vi "CalculateLowUpdateDeviceFeatures.vi"(8 "error in (no error)":errorcluster, 9 "data flow map in":T11, 10 "Waveforms":waveform(sgl)[](array[waveform]), 11 "Group in":T1={"Name"="", "Channels"=[], "Motor Information"={"Model"="", "Manufacturer"="", "Serial Number"="", "Horsepower"=0.0, "Horsepower Unit"="", "Full Load Speed"=0.0, "Synchronous Speed"=0.0, "Rated Volts"=0.0, "Full Load Amps"=0.0, "Frequency"=0.0, "Service Factor"=0.0, "Efficiency"=0.0, "Efficiency @ 75% Load"=0.0, "Efficiency @ 50% Load"=0.0, "Efficiency @ 25% Load"=0.0, "Power Factor"=0.0, "VoltageBus"="", "VoltageBus ID"="", "Stator Resistance"=0.0, "Estimate Stator Resistance"=FALSE}, "Calculation Cache"={"Spectrum Reset"=FALSE, "Spectrum"={"f0"=0.0, "df"=0.0, "magnitude [dB]"=[]}, "max sideband magnitude [dB]"=-100.0, "rotor sideband step [Hz]"=0.0, "spectrum initial conditions"={"hilbert state"={"delay conditions"=[], "filter conditions"=[]}, "zoom FFT state"={"phase state"=0.0, "zoom FFT state"={"zoom settings state"={"zoom"=0, "stop band attenuation"=enum."84 dB", "alias protect in final transition"=FALSE, "oversampling ratio"=0.0}, "SML Decimation Filter (complex input) state"={"decimation settings state"={"M"=0, "stop band attenuation"=enum."84 dB", "alias protect in transition band"=FALSE, "oversampling ratio"=0.0}, "counter for garbage samples state"=0, "sml_Parameter Setting for Zoom Factor state"={"filter length * interpolation state"=0, "interpolation state"=0, "comb filter order state"=0, "CFIR par state"={"h"=[], "M"=0, "N"=0}, "LFIR par state"={"h"=[], "M"=0, "N"=0}, "CIC Stages state"=0}, "aal_CIC (complex input) state"={"aal_cascaded moving average (complex input) state"={"states"=[], "circular buffers state"=[], "circular buffer counter state"=0}, "aal_moving average with decimation by order (complex input) state"={"residue result state"=0.0+0.0i, "processed data counter state"=0}}, "sml_Cascaded Decimation Filter (complex input) CFIR state"={"unprocessed data state"=[], "final conditions state"=[], "sml_M-1 Decimator with IC (complex input) state"={"coefficients in reverse order state"=[], "max index for coefficients state"=0}}, "sml_Cascaded Decimation Filter (complex input) LFIR state"={"unprocessed data state"=[], "final conditions state"=[], "sml_M-1 Decimator with IC (complex input) state"={"coefficients in reverse order state"=[], "max index for coefficients state"=0}}}, "ma_SML Data Packing (complex input) state"={"array getting packed state"=[], "last array processed state"=[], "index state"=0, "packing parameters state"={0, "size"=0}}}, "FFT{X} [Vrms]"=[]}, "IIR filter state"={"filter state"=[]}, "demodulation settings"={"enable? (F)"=FALSE, "algorithm"=enum."1-phase signal"}, "highpass IIR Filter"={"filter structure"=enum."IIR 2nd Order", "Reverse Coefficients"=[], "Forward Coefficients"=[]}, "Hilbert FIR filter"={"coefficients"=[], "delay"=0}, "zoom FFT settings"={"FFT settings"={"window"=0, "Window Size"=0, "FFT Size"=0, "%overlap"=0.0}, "zoom settings"={"zoom"=0, "stop band attenuation"=enum."84 dB", "alias protect in final transition"=FALSE, "oversampling ratio"=0.0}, "other settings"={"fmod"=0.0, "f0"=0.0, "df"=0.0, "oidx"=0, "olen"=0}, "iterations"=0, "max block size"=0, "fs"=0.0}}, "Speed Reset"=FALSE, "speed [RPM]"=0.0, "slip"=0.0, "speed initial conditions"={"SVAF state"={"space vector amplitude"=0.0, "hilbert state"={"delay conditions"=[], "filter conditions"=[]}}, "zoom FFT state"={"phase state"=0.0, "zoom FFT state"={"zoom settings state"={"zoom"=0, "stop band attenuation"=enum."84 dB", "alias protect in final transition"=FALSE, "oversampling ratio"=0.0}, "SML Decimation Filter (complex input) state"={"decimation settings state"={"M"=0, "stop band attenuation"=enum."84 dB", "alias protect in transition band"=FALSE, "oversampling ratio"=0.0}, "counter for garbage samples state"=0, "sml_Parameter Setting for Zoom Factor state"={"filter length * interpolation state"=0, "interpolation state"=0, "comb filter order state"=0, "CFIR par state"={"h"=[], "M"=0, "N"=0}, "LFIR par state"={"h"=[], "M"=0, "N"=0}, "CIC Stages state"=0}, "aal_CIC (complex input) state"={"aal_cascaded moving average (complex input) state"={"states"=[], "circular buffers state"=[], "circular buffer counter state"=0}, "aal_moving average with decimation by order (complex input) state"={"residue result state"=0.0+0.0i, "processed data counter state"=0}}, "sml_Cascaded Decimation Filter (complex input) CFIR state"={"unprocessed data state"=[], "final conditions state"=[], "sml_M-1 Decimator with IC (complex input) state"={"coefficients in reverse order state"=[], "max index for coefficients state"=0}}, "sml_Cascaded Decimation Filter (complex input) LFIR state"={"unprocessed data state"=[], "final conditions state"=[], "sml_M-1 Decimator with IC (complex input) state"={"coefficients in reverse order state"=[], "max index for coefficients state"=0}}}, "ma_SML Data Packing (complex input) state"={"array getting packed state"=[], "last array processed state"=[], "index state"=0, "packing parameters state"={0, "size"=0}}}, "FFT{X} [Vrms]"=[]}, "speed state"={"speed [RPM]"=0.0, "slip"=0.0}, "speed estimation settings"={"% overlap"=0.0, "algorithm"=enum."1-phase signal"}, "filter information"={"coefficients"=[], "order"=0}, "zoom FFT settings"={"FFT settings"={"window"=0, "Window Size"=0, "FFT Size"=0, "%overlap"=0.0}, "zoom settings"={"zoom"=0, "stop band attenuation"=enum."84 dB", "alias protect in final transition"=FALSE, "oversampling ratio"=0.0}, "other settings"={"fmod"=0.0, "f0"=0.0, "df"=0.0, "oidx"=0, "olen"=0}, "iterations"=0, "max block size"=0, "fs"=0.0}, "last valid window"=0, "fund. frequency for averager"=[]}, "line frequency [Hz]"=0.0}} {"Calculation Cache"."speed initial conditions"."zoom FFT settings"."FFT settings"."window" items=["Rectangle"=0, "Hanning"=1, "Hamming"=2, "Blackman-Harris"=3, "Exact Blackman"=4, "Blackman"=5, "Flat Top"=6, "4 Term B-Harris "=7, "7 Term B-Harris"=8, "Low Sidelobe"=9, "Blackman Nuttall"=11, "Triangle"=30, "Bartlett-Hanning"=31, "Bohman"=32, "Parzen"=33, "Welch"=34, "Kaiser"=60, "Dolph-Chebyshev"=61, "Gaussian"=62]; "Calculation Cache"."spectrum initial conditions"."zoom FFT settings"."FFT settings"."window" items=["Rectangle"=0, "Hanning"=1, "Hamming"=2, "Blackman-Harris"=3, "Exact Blackman"=4, "Blackman"=5, "Flat Top"=6, "4 Term B-Harris "=7, "7 Term B-Harris"=8, "Low Sidelobe"=9, "Blackman Nuttall"=11, "Triangle"=30, "Bartlett-Hanning"=31, "Bohman"=32, "Parzen"=33, "Welch"=34, "Kaiser"=60, "Dolph-Chebyshev"=61, "Gaussian"=62]}) -> (0 "error out":errorcluster, 3 "Group out":T1={"Name"="", "Channels"=[], "Motor Information"={"Model"="", "Manufacturer"="", "Serial Number"="", "Horsepower"=0.0, "Horsepower Unit"="", "Full Load Speed"=0.0, "Synchronous Speed"=0.0, "Rated Volts"=0.0, "Full Load Amps"=0.0, "Frequency"=0.0, "Service Factor"=0.0, "Efficiency"=0.0, "Efficiency @ 75% Load"=0.0, "Efficiency @ 50% Load"=0.0, "Efficiency @ 25% Load"=0.0, "Power Factor"=0.0, "VoltageBus"="", "VoltageBus ID"="", "Stator Resistance"=0.0, "Estimate Stator Resistance"=FALSE}, "Calculation Cache"={"Spectrum Reset"=FALSE, "Spectrum"={"f0"=0.0, "df"=0.0, "magnitude [dB]"=[]}, "max sideband magnitude [dB]"=-100.0, "rotor sideband step [Hz]"=0.0, "spectrum initial conditions"={"hilbert state"={"delay conditions"=[], "filter conditions"=[]}, "zoom FFT state"={"phase state"=0.0, "zoom FFT state"={"zoom settings state"={"zoom"=0, "stop band attenuation"=enum."84 dB", "alias protect in final transition"=FALSE, "oversampling ratio"=0.0}, "SML Decimation Filter (complex input) state"={"decimation settings state"={"M"=0, "stop band attenuation"=enum."84 dB", "alias protect in transition band"=FALSE, "oversampling ratio"=0.0}, "counter for garbage samples state"=0, "sml_Parameter Setting for Zoom Factor state"={"filter length * interpolation state"=0, "interpolation state"=0, "comb filter order state"=0, "CFIR par state"={"h"=[], "M"=0, "N"=0}, "LFIR par state"={"h"=[], "M"=0, "N"=0}, "CIC Stages state"=0}, "aal_CIC (complex input) state"={"aal_cascaded moving average (complex input) state"={"states"=[], "circular buffers state"=[], "circular buffer counter state"=0}, "aal_moving average with decimation by order (complex input) state"={"residue result state"=0.0+0.0i, "processed data counter state"=0}}, "sml_Cascaded Decimation Filter (complex input) CFIR state"={"unprocessed data state"=[], "final conditions state"=[], "sml_M-1 Decimator with IC (complex input) state"={"coefficients in reverse order state"=[], "max index for coefficients state"=0}}, "sml_Cascaded Decimation Filter (complex input) LFIR state"={"unprocessed data state"=[], "final conditions state"=[], "sml_M-1 Decimator with IC (complex input) state"={"coefficients in reverse order state"=[], "max index for coefficients state"=0}}}, "ma_SML Data Packing (complex input) state"={"array getting packed state"=[], "last array processed state"=[], "index state"=0, "packing parameters state"={0, "size"=0}}}, "FFT{X} [Vrms]"=[]}, "IIR filter state"={"filter state"=[]}, "demodulation settings"={"enable? (F)"=FALSE, "algorithm"=enum."1-phase signal"}, "highpass IIR Filter"={"filter structure"=enum."IIR 2nd Order", "Reverse Coefficients"=[], "Forward Coefficients"=[]}, "Hilbert FIR filter"={"coefficients"=[], "delay"=0}, "zoom FFT settings"={"FFT settings"={"window"=0, "Window Size"=0, "FFT Size"=0, "%overlap"=0.0}, "zoom settings"={"zoom"=0, "stop band attenuation"=enum."84 dB", "alias protect in final transition"=FALSE, "oversampling ratio"=0.0}, "other settings"={"fmod"=0.0, "f0"=0.0, "df"=0.0, "oidx"=0, "olen"=0}, "iterations"=0, "max block size"=0, "fs"=0.0}}, "Speed Reset"=FALSE, "speed [RPM]"=0.0, "slip"=0.0, "speed initial conditions"={"SVAF state"={"space vector amplitude"=0.0, "hilbert state"={"delay conditions"=[], "filter conditions"=[]}}, "zoom FFT state"={"phase state"=0.0, "zoom FFT state"={"zoom settings state"={"zoom"=0, "stop band attenuation"=enum."84 dB", "alias protect in final transition"=FALSE, "oversampling ratio"=0.0}, "SML Decimation Filter (complex input) state"={"decimation settings state"={"M"=0, "stop band attenuation"=enum."84 dB", "alias protect in transition band"=FALSE, "oversampling ratio"=0.0}, "counter for garbage samples state"=0, "sml_Parameter Setting for Zoom Factor state"={"filter length * interpolation state"=0, "interpolation state"=0, "comb filter order state"=0, "CFIR par state"={"h"=[], "M"=0, "N"=0}, "LFIR par state"={"h"=[], "M"=0, "N"=0}, "CIC Stages state"=0}, "aal_CIC (complex input) state"={"aal_cascaded moving average (complex input) state"={"states"=[], "circular buffers state"=[], "circular buffer counter state"=0}, "aal_moving average with decimation by order (complex input) state"={"residue result state"=0.0+0.0i, "processed data counter state"=0}}, "sml_Cascaded Decimation Filter (complex input) CFIR state"={"unprocessed data state"=[], "final conditions state"=[], "sml_M-1 Decimator with IC (complex input) state"={"coefficients in reverse order state"=[], "max index for coefficients state"=0}}, "sml_Cascaded Decimation Filter (complex input) LFIR state"={"unprocessed data state"=[], "final conditions state"=[], "sml_M-1 Decimator with IC (complex input) state"={"coefficients in reverse order state"=[], "max index for coefficients state"=0}}}, "ma_SML Data Packing (complex input) state"={"array getting packed state"=[], "last array processed state"=[], "index state"=0, "packing parameters state"={0, "size"=0}}}, "FFT{X} [Vrms]"=[]}, "speed state"={"speed [RPM]"=0.0, "slip"=0.0}, "speed estimation settings"={"% overlap"=0.0, "algorithm"=enum."1-phase signal"}, "filter information"={"coefficients"=[], "order"=0}, "zoom FFT settings"={"FFT settings"={"window"=0, "Window Size"=0, "FFT Size"=0, "%overlap"=0.0}, "zoom settings"={"zoom"=0, "stop band attenuation"=enum."84 dB", "alias protect in final transition"=FALSE, "oversampling ratio"=0.0}, "other settings"={"fmod"=0.0, "f0"=0.0, "df"=0.0, "oidx"=0, "olen"=0}, "iterations"=0, "max block size"=0, "fs"=0.0}, "last valid window"=0, "fund. frequency for averager"=[]}, "line frequency [Hz]"=0.0}} {"Calculation Cache"."speed initial conditions"."zoom FFT settings"."FFT settings"."window" items=["Rectangle"=0, "Hanning"=1, "Hamming"=2, "Blackman-Harris"=3, "Exact Blackman"=4, "Blackman"=5, "Flat Top"=6, "4 Term B-Harris "=7, "7 Term B-Harris"=8, "Low Sidelobe"=9, "Blackman Nuttall"=11, "Triangle"=30, "Bartlett-Hanning"=31, "Bohman"=32, "Parzen"=33, "Welch"=34, "Kaiser"=60, "Dolph-Chebyshev"=61, "Gaussian"=62]; "Calculation Cache"."spectrum initial conditions"."zoom FFT settings"."FFT settings"."window" items=["Rectangle"=0, "Hanning"=1, "Hamming"=2, "Blackman-Harris"=3, "Exact Blackman"=4, "Blackman"=5, "Flat Top"=6, "4 Term B-Harris "=7, "7 Term B-Harris"=8, "Low Sidelobe"=9, "Blackman Nuttall"=11, "Triangle"=30, "Bartlett-Hanning"=31, "Bohman"=32, "Parzen"=33, "Welch"=34, "Kaiser"=60, "Dolph-Chebyshev"=61, "Gaussian"=62]})   [LabVIEW 2017, in "McsaAnalysisLowUpdate.lvlib"]
uses:
  <vilib>/addons/InsightCM/Devices/Shared/Mcsa/McsaAnalysisLowUpdate/McsaAnalysisLowUpdate.lvlib
  <vilib>/addons/PointValueMap/controls/PointMap.ctl
  <vilib>/addons/InsightCM/Devices/Shared/Mcsa/McsaAnalysisLowUpdate/controls/Group.ctl
  <vilib>/addons/InsightCM/Utilities/Analysis/MCSA/controls/McsaLowUpdateChannel.ctl
  <vilib>/addons/InsightCM/Utilities/Analysis/Shared/controls/Feature.ctl
  <vilib>/addons/InsightCM/Utilities/Analysis/Shared/controls/AmplitudeScale.ctl
  <vilib>/addons/InsightCM/Utilities/Analysis/MCSA/controls/McsaMotor.ctl
  <vilib>/addons/InsightCM/Utilities/Analysis/MCSA/controls/McsaCalculationCache.ctl
  <vilib>/addons/Electrical Power/Motor Monitoring/subVIs/ep_Initial Conditions for MCSA Spectra.ctl
  <vilib>/addons/Electrical Power/Motor Monitoring/subVIs/ep_Demodulation Algorithm.ctl
  <vilib>/addons/Electrical Power/Motor Monitoring/subVIs/ep_Zoom FFT Settings.ctl
  <vilib>/addons/Electrical Power/Motor Monitoring/subVIs/ep_Initial Conditions for Speed Estimation.ctl
  <vilib>/addons/InsightCM/Utilities/Analysis/MCSA/McsaAnalysisFunctions.lvlib
  <vilib>/addons/PointValueMap/PointValueMap.lvlib
  <vilib>/addons/InsightCM/Utilities/Analysis/Shared/AnalysisHelper.lvlib
  <vilib>/addons/Electrical Power/Motor Monitoring/NI_EP_Motor Monitoring.lvlib
panel:
  out "data flow map out":T11
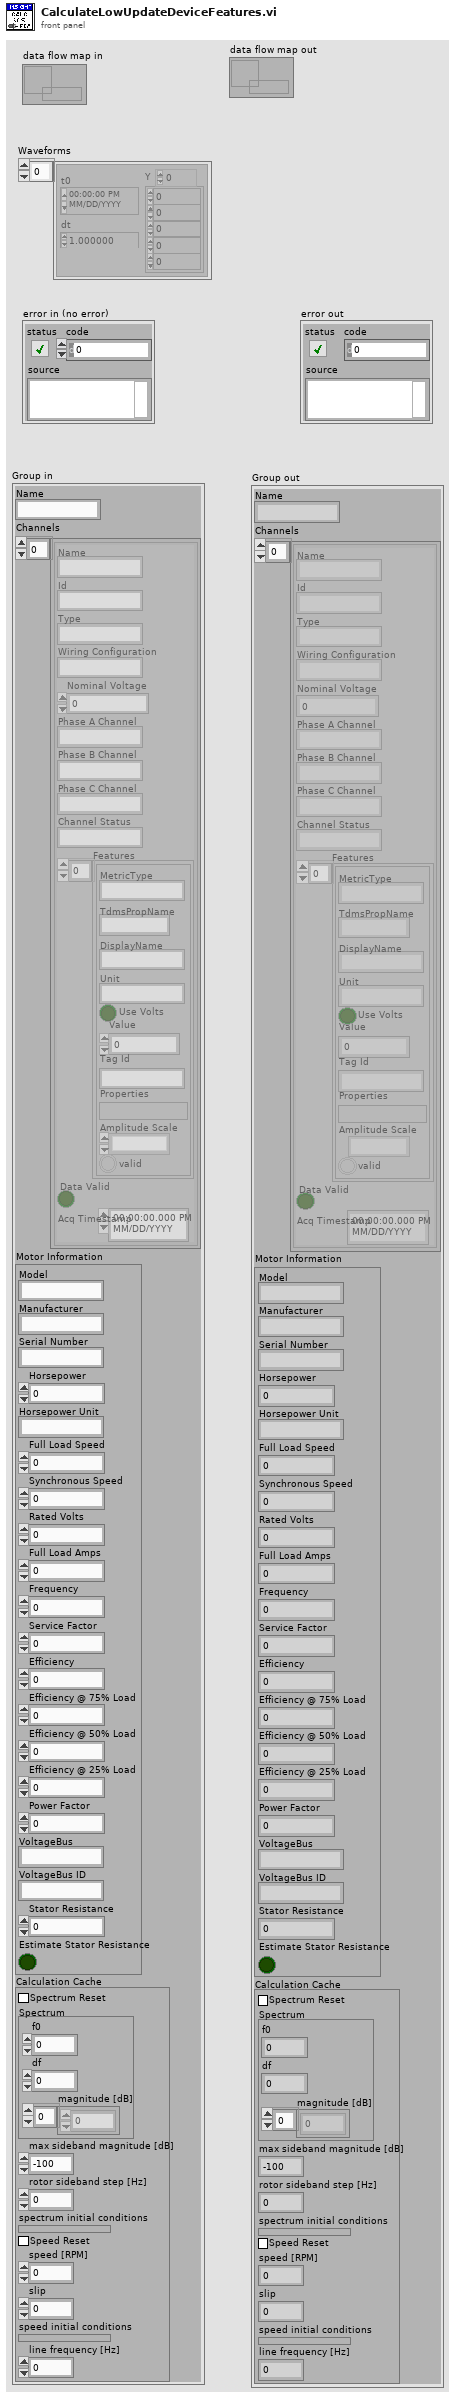
[diagram p1: front panel]
types:
  T1 = typedef "McsaAnalysisLowUpdate.lvlib/Group.ctl" = cluster{"Name":string, "Channels":T2[], "Motor Information":T5, "Calculation Cache":T6}
  T2 = typedef "McsaAnalysisFunctions.lvlib/McsaLowUpdateChannel.ctl" = cluster{"Name":string, "Id":string, "Type":string, "Wiring Configuration":string, "Nominal Voltage":dbl, "Phase A Channel":string, "Phase B Channel":string, "Phase C Channel":string, "Channel Status":string, "Features":T3[], "Data Valid":bool, "Acq Timestamp":timestamp}
  T3 = typedef "AnalysisHelper.lvlib/Feature.ctl" = cluster{"MetricType":string, "TdmsPropName":string, "DisplayName":string, "Unit":string, "Use Volts":bool, "Value":dbl, "Tag Id":string, "Properties":variant, "Amplitude Scale":T4, "valid":bool}
  T4 = typedef "AnalysisHelper.lvlib/AmplitudeScale.ctl" = enum16{"rms", "peak", "pk-pk"}
  T5 = typedef "McsaAnalysisFunctions.lvlib/McsaMotor.ctl" = cluster{"Model":string, "Manufacturer":string, "Serial Number":string, "Horsepower":dbl, "Horsepower Unit":string, "Full Load Speed":dbl, "Synchronous Speed":dbl, "Rated Volts":dbl, "Full Load Amps":dbl, "Frequency":dbl, "Service Factor":dbl, "Efficiency":dbl, "Efficiency @ 75% Load":dbl, "Efficiency @ 50% Load":dbl, "Efficiency @ 25% Load":dbl, "Power Factor":dbl, "VoltageBus":string, "VoltageBus ID":string, "Stator Resistance":dbl, "Estimate Stator Resistance":bool}
  T6 = typedef "McsaAnalysisFunctions.lvlib/McsaCalculationCache.ctl" = cluster{"Spectrum Reset":bool, "Spectrum":cluster{"f0":dbl, "df":dbl, "magnitude [dB]":dbl[]}, "max sideband magnitude [dB]":dbl, "rotor sideband step [Hz]":dbl, "spectrum initial conditions":T7, "Speed Reset":bool, "speed [RPM]":dbl, "slip":dbl, "speed initial conditions":T10, "line frequency [Hz]":dbl}
  T7 = typedef "NI_EP_Motor Monitoring.lvlib/ep_Initial Conditions for MCSA Spectra.ctl" = cluster{"hilbert state":cluster{"delay conditions":dbl[], "filter conditions":dbl[]}, "zoom FFT state":cluster{"phase state":dbl, "zoom FFT state":cluster{"zoom settings state":cluster{"zoom":i32, "stop band attenuation":enum16{"84 dB", "96 dB", "120 dB"}, "alias protect in final transition":bool, "oversampling ratio":dbl}, "SML Decimation Filter (complex input) state":cluster{"decimation settings state":cluster{"M":i32, "stop band attenuation":enum16{"84 dB", "96 dB", "120 dB"}, "alias protect in transition band":bool, "oversampling ratio":dbl}, "counter for garbage samples state":i32, "sml_Parameter Setting for Zoom Factor state":cluster{"filter length * interpolation state":i32, "interpolation state":i32, "comb filter order state":i32, "CFIR par state":cluster{"h":dbl[], "M":i32, "N":i32}, "LFIR par state":cluster{"h":dbl[], "M":i32, "N":i32}, "CIC Stages state":i32}, "aal_CIC (complex input) state":cluster{"aal_cascaded moving average (complex input) state":cluster{"states":cdb[], "circular buffers state":cdb[][], "circular buffer counter state":i32}, "aal_moving average with decimation by order (complex input) state":cluster{"residue result state":cdb, "processed data counter state":i32}}, "sml_Cascaded Decimation Filter (complex input) CFIR state":cluster{"unprocessed data state":cdb[], "final conditions state":cdb[][], "sml_M-1 Decimator with IC (complex input) state":cluster{"coefficients in reverse order state":dbl[], "max index for coefficients state":i32}}, "sml_Cascaded Decimation Filter (complex input) LFIR state":cluster{"unprocessed data state":cdb[], "final conditions state":cdb[][], "sml_M-1 Decimator with IC (complex input) state":cluster{"coefficients in reverse order state":dbl[], "max index for coefficients state":i32}}}, "ma_SML Data Packing (complex input) state":cluster{"array getting packed state":cdb[], "last array processed state":cdb[], "index state":i32, "packing parameters state":cluster{i32, "size":i32}}}, "FFT{X} [Vrms]":cdb[]}, "IIR filter state":cluster{"filter state":dbl[]}, "demodulation settings":cluster{"enable? (F)":bool, "algorithm":T8}, "highpass IIR Filter":cluster{"filter structure":enum32{"IIR 2nd Order", "IIR 4th Order"}, "Reverse Coefficients":dbl[], "Forward Coefficients":dbl[]}, "Hilbert FIR filter":cluster{"coefficients":dbl[], "delay":i32}, "zoom FFT settings":T9}
  T8 = typedef "NI_EP_Motor Monitoring.lvlib/ep_Demodulation Algorithm.ctl" = enum16{"1-phase signal", "3-phase signals"}
  T9 = typedef "NI_EP_Motor Monitoring.lvlib/ep_Zoom FFT Settings.ctl" = cluster{"FFT settings":cluster{"window":u16, "Window Size":i32, "FFT Size":i32, "%overlap":dbl}, "zoom settings":cluster{"zoom":i32, "stop band attenuation":enum16{"84 dB", "96 dB", "120 dB"}, "alias protect in final transition":bool, "oversampling ratio":dbl}, "other settings":cluster{"fmod":dbl, "f0":dbl, "df":dbl, "oidx":i32, "olen":i32}, "iterations":i32, "max block size":i32, "fs":dbl}
  T10 = typedef "NI_EP_Motor Monitoring.lvlib/ep_Initial Conditions for Speed Estimation.ctl" = cluster{"SVAF state":cluster{"space vector amplitude":dbl, "hilbert state":cluster{"delay conditions":dbl[], "filter conditions":dbl[]}}, "zoom FFT state":cluster{"phase state":dbl, "zoom FFT state":cluster{"zoom settings state":cluster{"zoom":i32, "stop band attenuation":enum16{"84 dB", "96 dB", "120 dB"}, "alias protect in final transition":bool, "oversampling ratio":dbl}, "SML Decimation Filter (complex input) state":cluster{"decimation settings state":cluster{"M":i32, "stop band attenuation":enum16{"84 dB", "96 dB", "120 dB"}, "alias protect in transition band":bool, "oversampling ratio":dbl}, "counter for garbage samples state":i32, "sml_Parameter Setting for Zoom Factor state":cluster{"filter length * interpolation state":i32, "interpolation state":i32, "comb filter order state":i32, "CFIR par state":cluster{"h":dbl[], "M":i32, "N":i32}, "LFIR par state":cluster{"h":dbl[], "M":i32, "N":i32}, "CIC Stages state":i32}, "aal_CIC (complex input) state":cluster{"aal_cascaded moving average (complex input) state":cluster{"states":cdb[], "circular buffers state":cdb[][], "circular buffer counter state":i32}, "aal_moving average with decimation by order (complex input) state":cluster{"residue result state":cdb, "processed data counter state":i32}}, "sml_Cascaded Decimation Filter (complex input) CFIR state":cluster{"unprocessed data state":cdb[], "final conditions state":cdb[][], "sml_M-1 Decimator with IC (complex input) state":cluster{"coefficients in reverse order state":dbl[], "max index for coefficients state":i32}}, "sml_Cascaded Decimation Filter (complex input) LFIR state":cluster{"unprocessed data state":cdb[], "final conditions state":cdb[][], "sml_M-1 Decimator with IC (complex input) state":cluster{"coefficients in reverse order state":dbl[], "max index for coefficients state":i32}}}, "ma_SML Data Packing (complex input) state":cluster{"array getting packed state":cdb[], "last array processed state":cdb[], "index state":i32, "packing parameters state":cluster{i32, "size":i32}}}, "FFT{X} [Vrms]":cdb[]}, "speed state":cluster{"speed [RPM]":dbl, "slip":dbl}, "speed estimation settings":cluster{"% overlap":dbl, "algorithm":T8}, "filter information":cluster{"coefficients":dbl[], "order":i32}, "zoom FFT settings":T9, "last valid window":i32, "fund. frequency for averager":dbl[]}
  T11 = typedef "PointValueMap.lvlib/PointMap.ctl" = refnum<data-value>
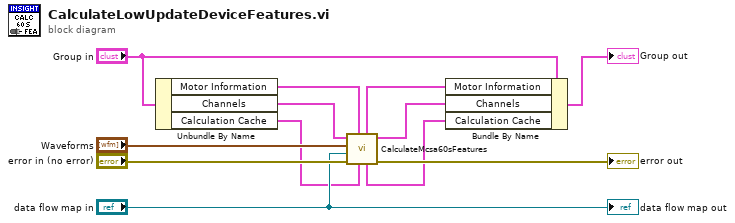
[diagram p0: block diagram]
diagram:
  n1 = Unbundle By Name("Group in") -> ("Motor Information"=w7:T5, "Channels"=w8:T2[], "Calculation Cache"=w6:T6)
  n2 = call <vilib>:"CalculateMcsa60sFeatures.vi"("Calculation Cache"=w6, "Motor Information"=w7, "error in (no error)"="error in (no error)", "data flow map in"="data flow map in", "waveforms"="Waveforms", "Channels"=w8) -> ("error out"=→"error out":errorcluster, "Channels out"=w3:T2[], "Calculation Cache out"=w2:T6, "Motor Information out"=w4:T5)  [unwired: 2 in]
  n3 = Bundle By Name(cluster="Group in", "Motor Information"=w4, "Channels"=w3, "Calculation Cache"=w2) -> (→"Group out":T1)
  "data flow map out" <- "data flow map in"
